vi "Generate_Signals.vi"() -> ()   [LabVIEW 2016]
uses:
  <vilib>/Analysis/NI_AALBase.lvlib
panel:
  out "Output":string
  out "error out":errorcluster
  in  "Filename":string="GeneratedSignals"
  in  "Output destination":path=path "C:/Users/Erwin/Desktop"
  out "Waveform Graph":u16[][](graph)
  in  "amplitude":u16=4096
  in  "Number of Samples":i32=64
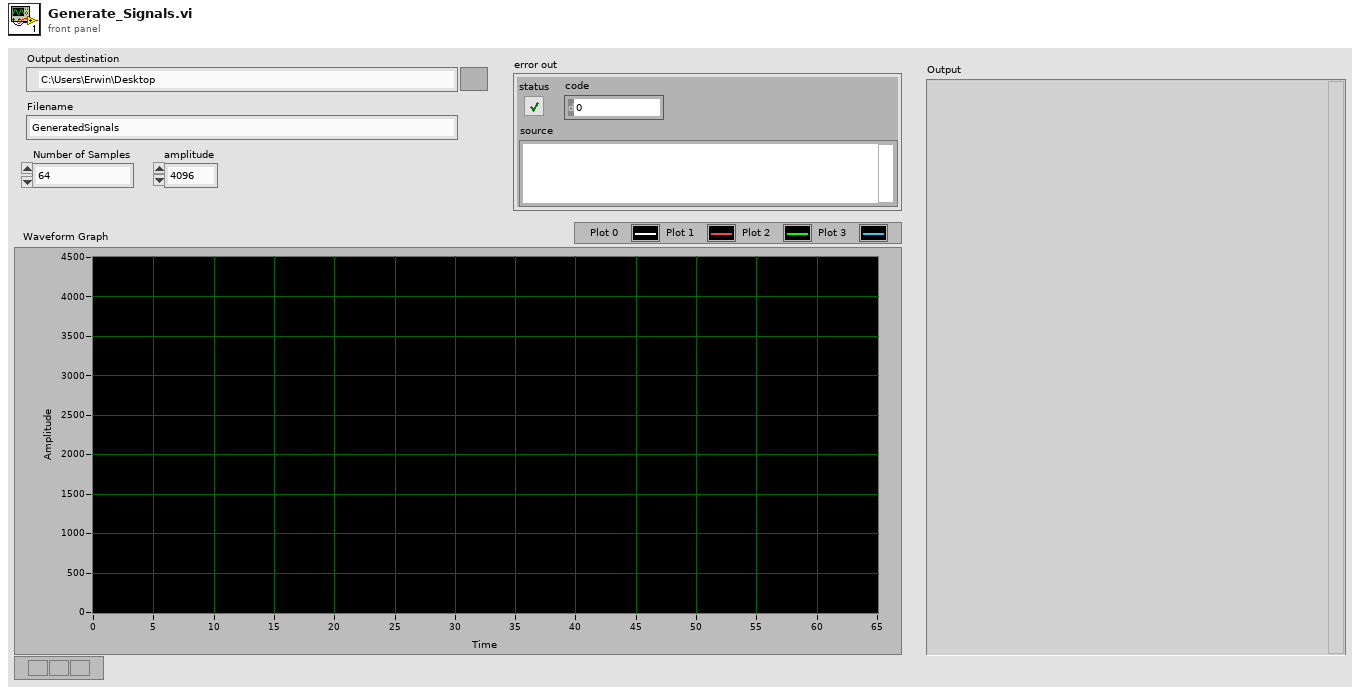
[diagram p1: front panel]
types:
  T1 = enum16{"open", "replace", "create", "open or create", "replace or create", "replace or create with confirmation"}
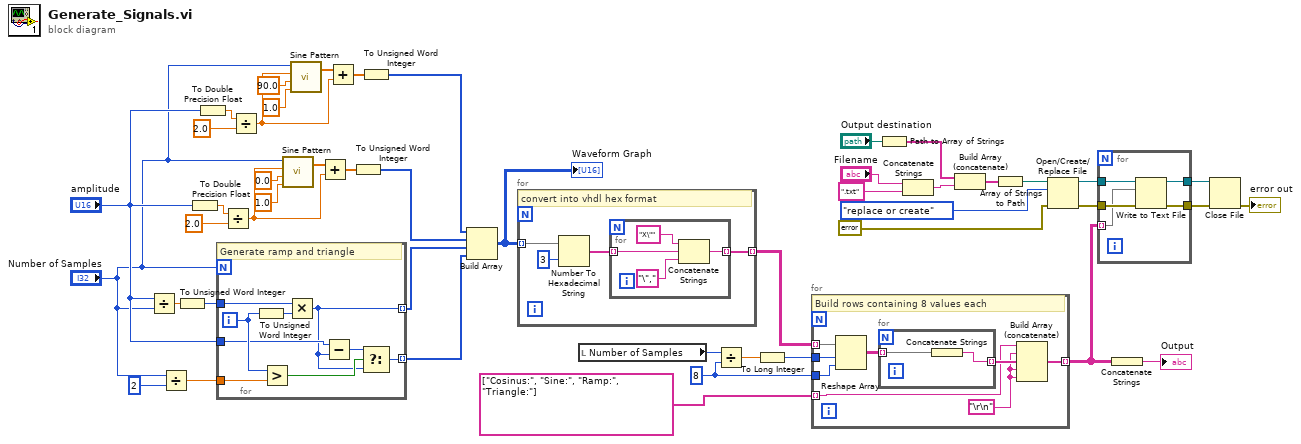
[diagram p0: block diagram]
diagram:
  w18 = 8 ("dimension size")
  n1 = Divide(x="amplitude", y="Number of Samples") -> (x/y=w39:dbl)
  n2 = Divide(x="Number of Samples", y=2 ("x")) -> (x/y=w15:dbl)
  n3 = To Unsigned Word Integer(number=w39) -> (unsigned 16bit integer=w16:u16)
  n4 = To Double Precision Float(number="amplitude") -> (double precision float=w41:dbl)
  n5 = To Double Precision Float(number="amplitude") -> (double precision float=w10:dbl)
  n6 = for {
    N: "Number of Samples" -> [_]
    tunnel: w16 -> [w56]
    tunnel: [w48] -> w38 mode=indexing
    tunnel: w15 -> [w53]
    tunnel: "amplitude" -> [w52]
    tunnel: [w50] -> w13 mode=indexing
    i -> [w54]
    # "Generate ramp and triangle"
    n7 = To Unsigned Word Integer(number=w54) -> (unsigned 16bit integer=w55:u16)
    n8 = Greater?(x=w54, y=w53) -> (0:w49:bool)
    n9 = Multiply(x=w56, y=w55) -> (x*y=w48:u16)
    n10 = Subtract(x=w52, y=w48) -> (x-y=w51:u16)
    n11 = Select(t=w51, s=w49, f=w48) -> (s? t:f=w50:u16)
  }
  n12 = Divide(x=w41, y=2.0) -> (x/y=w44:dbl)
  n13 = Divide(x=w10, y=2.0) -> (x/y=w7:dbl)
  n14 = call <vilib>:"Sine Pattern.vi"("cycles"=1.0, "phase(degrees)"=0.0, "amplitude"=w44, "samples"="Number of Samples") -> ("Sinusoidal Pattern"=w45:dbl[])  [unwired: 1 out]
  n15 = call <vilib>:"Sine Pattern.vi"("cycles"=1.0, "phase(degrees)"=90.0, "amplitude"=w7, "samples"="Number of Samples") -> ("Sinusoidal Pattern"=w6:dbl[])  [unwired: 1 out]
  n16 = Add(x=w45, y=w44) -> (x+y=w43:dbl[])
  n17 = Add(x=w6, y=w7) -> (x+y=w8:dbl[])
  n18 = To Unsigned Word Integer(number=w43) -> (unsigned 16bit integer=w40:u16[])
  n19 = To Unsigned Word Integer(number=w8) -> (unsigned 16bit integer=w1:u16[])
  n20 = Build Array(w1, w40, w38, w13) -> (w37:u16[][])
  "Waveform Graph" <- w37
  n21 = for {
    tunnel: w37 -> [w58] mode=indexing
    tunnel: [w57] -> w22 mode=indexing
    # "convert into vhdl hex format"
    n22 = Number To Hexadecimal String(1:i16 3 ("width (-)"), 2:w58) -> (0:w59:string[])
    n23 = for {
      tunnel: w59 -> [w64] mode=indexing
      tunnel: [w61] -> w57 mode=indexing
      n24 = Concatenate Strings("X\"" ("string"), w64, "\"," ("string")) -> (w61:string)
    }
  }
  n25 = local read "Number of Samples"() -> (w21:i32)
  n26 = Divide(x=w21, y=w18) -> (x/y=w20:dbl)
  n27 = To Long Integer(number=w20) -> (32bit integer=w19:i32)
  n28 = for {
    tunnel: w22 -> [w72] mode=indexing
    tunnel: w19 -> [w71]
    tunnel: w18 -> [w70]
    tunnel: [w67] -> w11 mode=indexing
    tunnel: string[] ["Cosinus:", "Sine:", "Ramp:", "Triangle:"] -> [w66] mode=indexing
    w65 = "\r\n"
    # "Build rows containing 8 values each"
    n29 = Reshape Array(w72, w71, w70) -> (w69:string[][])
    n30 = for {
      tunnel: w69 -> [w74] mode=indexing
      tunnel: [w73] -> w68 mode=indexing
      n31 = Concatenate Strings(w74) -> (w73:string)
    }
    n32 = Build Array (concatenate)(w66, w65, w68, w65, w65) -> (w67:string[])
  }
  n33 = Path to Array of Strings(0:"Output destination") -> (2:w33:string[])  [unwired: 1 out]
  n34 = Concatenate Strings("Filename", ".txt" ("string")) -> (w24:string)
  n35 = Build Array (concatenate)(w33, w24) -> (w31:string[])
  n36 = Array of Strings to Path(0:w31) -> (2:w30:path)  [unwired: 1 in]
  n37 = Open/Create/Replace File(file path (use dialog)=w30, error in=errorcluster {"status"=FALSE, "code"=0, "source"=""}, operation (0:open)=T1."replace or create") -> (refnum out=w36:refnum<file>, error out=w35:errorcluster)  [unwired: 3 in, 1 out]
  n38 = for {
    tunnel: w36 -> [w79]
    tunnel: w35 -> [w78]
    tunnel: w11 -> [w77] mode=indexing
    tunnel: [w76] -> w28
    tunnel: [w75] -> w27
    n39 = Write to Text File(file (use dialog)=w79, text=w77, error in=w78) -> (refnum out=w76:refnum<file>, error out=w75:errorcluster)  [unwired: 1 in, 1 out]
  }
  n40 = Concatenate Strings(w11) -> (→"Output":string)
  n41 = Close File(refnum=w28, error in=w27) -> (error out=→"error out":errorcluster)  [unwired: 1 out]
